vi "ForebrainMain.vi"() -> ()   [LabVIEW 2012]
uses:
  <vilib>/Utility/inputDevices.llb/closeKeyboard.vi
  <vilib>/Utility/inputDevices.llb/keyboardAcquire.vi
panel:
  out "IR Data":dbl
  in  "Send to XBEE":string
  out "bytes written":u32
  out "Sent from XBEE":string
  out "return count":u32
  out "XBEE Working":bool
  in  "FULL STOP":bool
  in  "PC Status":i32=1
  out "Port Rudder":i32
  out "Starboard Rudder":i32
  out "Port Motor":i32
  out "Starboard Motor":i32
  in  "VISA resource name":refnum<visa-resource-name>="COM6"
  in  "error in":errorcluster
  out "Base Station data rec'd":string
  out "Robot Stats":i32[](array[numeric])
  out "Buoy locations":cluster{"regular expression":string, i32, i32}[](array[cluster])
  in  "Tab Control":T1(tab)
  in  "End Rc Session":bool
  in  "Pan Camera":i32(slide)=1500 scale=500.0..2500.0
  in  "MANUAL \nOVERRIDE":bool
  out "Speed                    Balance":i32(knob) scale=-1000.0..1000.0
  in  "Step Size":i32=5
  in  "Rudders":i32(slide)=1500 scale=500.0..2500.0
  out "Port Speed":i32(knob) scale=1000.0..2000.0
  out "Starboard Speed":i32(knob) scale=1000.0..2000.0
  out "Obstacle Seen":bool
  in  "Launch":bool
  out "Forward":u8(slide) scale=0.0..100.0
  in  "Mission Selection":string(combo)
  out "Backward":u8(slide) scale=0.0..100.0
  # "This is the main VI.\n\nThis will allow you to debug the sensor system, remotely control the boat, and select a mission for the boat to run autonomously.  This code will connect to the base station, use the XBEE to connect to the boat, and use Labview as an interfacing platform with the boat.\n\nIf you have questions/comments/concerns, email Bill Warner or Victoria Preston (Olin)\n\nCreated:Feb 28, 2014\nRevised: Mar 9, 2014"
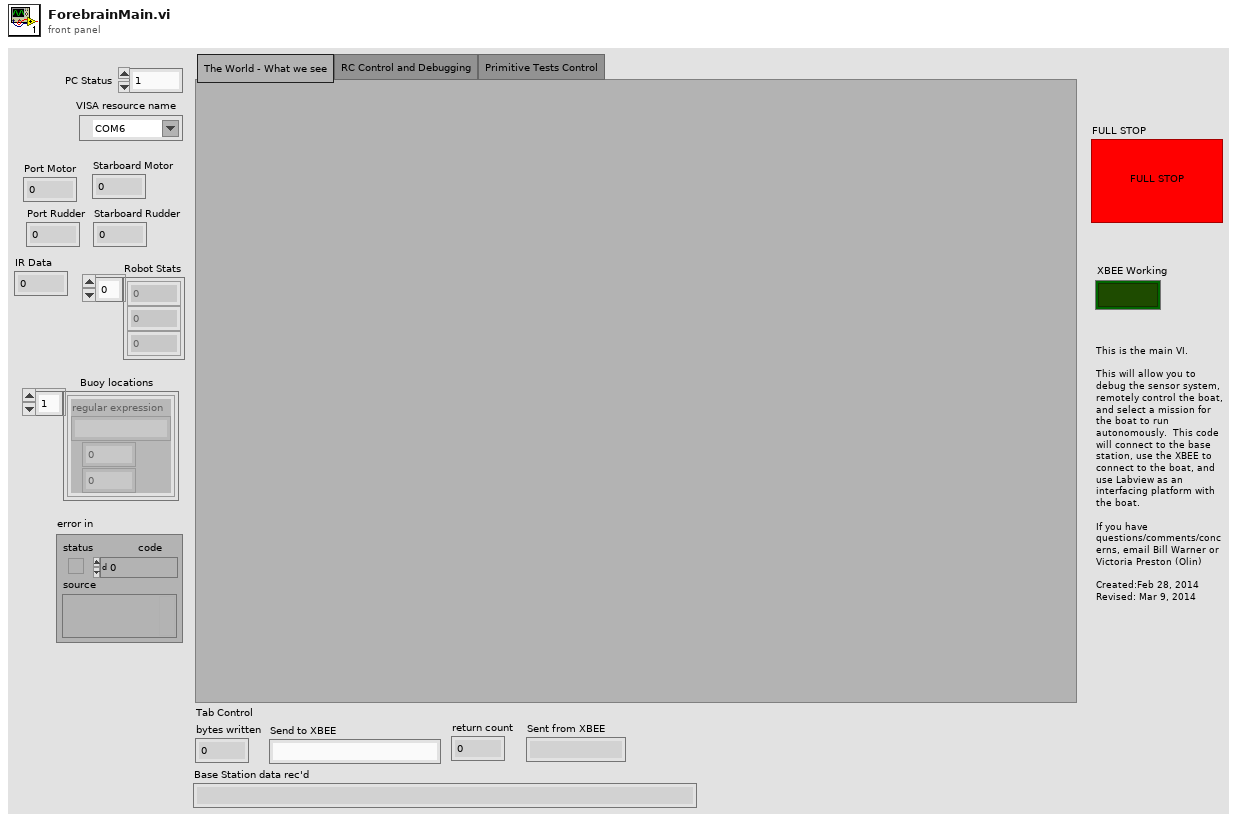
[diagram p1: front panel]
types:
  T1 = enum32{"The World - What we see", "RC Control and Debugging", "Primitive Tests Control"}
  T2 = enum16{"0", "1", "2", "3", "4", "5", "6", "7", "8", "9", "A", "B", "C", "D", "E", "F", "G", "H", "I", "J", "K", "L", "M", "N", "O", "P", "Q", "R", "S", "T", "U", "V", "W", "X", "Y", "Z", "F1", "F2", "F3", "F4", "F5", "F6", "F7", "F8", "F9", "F10", "F11", "F12", "F13", "F14", "F15", "ADD", "BACK", "BACKSLASH", "CAPITAL", "COMMA", "DECIMAL", "DELETE", "DIVIDE", "DOWN", "END", "EQUALS", "ESCAPE", "GRAVE (`)", "HOME", "INSERT", "LBRACKET", "LCONTROL", "LEFT", "L ALT", "LSHIFT", "LWIN", "MINUS", "MULTIPLY", "NEXT", "NUMLOCK", "NUMPAD_0", "NUMPAD_1", "NUMPAD_2", "NUMPAD_3", "NUMPAD_4", "NUMPAD_5", "NUMPAD_6", "NUMPAD_7", "NUMPAD_8", "NUMPAD_9", "PAUSE", "PERIOD", "PRIOR (PG UP)", "RBRACKET", "RCONTROL", "RETURN", "RIGHT", "R ALT", "RSHIFT", "RWIN", "SCROLL", "SEMICOLON", "SLASH", "SPACE", "SUBTRACT", "TAB", "UP", "ENTER (num pad)", "' (quote)"}[]
  T3 = enum16{"0", "1", "2", "3", "4", "5", "6", "7", "8", "9", "A", "B", "C", "D", "E", "F", "G", "H", "I", "J", "K", "L", "M", "N", "O", "P", "Q", "R", "S", "T", "U", "V", "W", "X", "Y", "Z", "F1", "F2", "F3", "F4", "F5", "F6", "F7", "F8", "F9", "F10", "F11", "F12", "F13", "F14", "F15", "ADD", "BACK", "BACKSLASH", "CAPITAL", "COMMA", "DECIMAL", "DELETE", "DIVIDE", "DOWN", "END", "EQUALS", "ESCAPE", "GRAVE (`)", "HOME", "INSERT", "LBRACKET", "LCONTROL", "LEFT", "L ALT", "LSHIFT", "LWIN", "MINUS", "MULTIPLY", "NEXT", "NUMLOCK", "NUMPAD_0", "NUMPAD_1", "NUMPAD_2", "NUMPAD_3", "NUMPAD_4", "NUMPAD_5", "NUMPAD_6", "NUMPAD_7", "NUMPAD_8", "NUMPAD_9", "PAUSE", "PERIOD", "PRIOR (PG UP)", "RBRACKET", "RCONTROL", "RETURN", "RIGHT", "R ALT", "RSHIFT", "RWIN", "SCROLL", "SEMICOLON", "SLASH", "SPACE", "SUBTRACT", "TAB", "UP", "ENTER (num pad)", "' (quote)"}
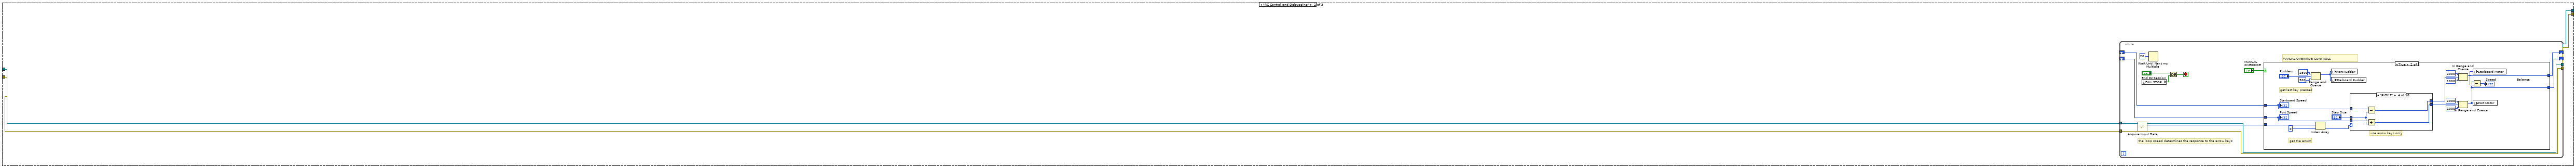
[diagram p3: hidden frame]
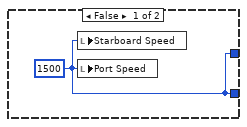
[diagram p4: hidden frame]
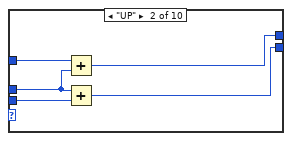
[diagram p6: hidden frame]
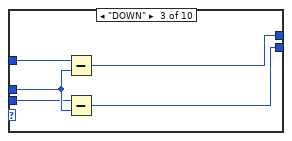
[diagram p7: hidden frame]
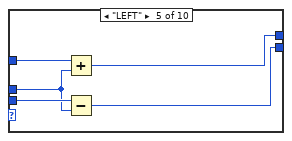
[diagram p8: hidden frame]
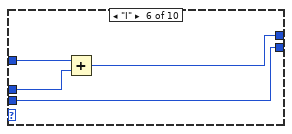
[diagram p9: hidden frame]
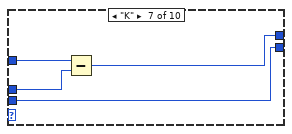
[diagram p10: hidden frame]
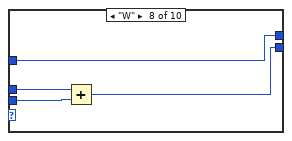
[diagram p11: hidden frame]
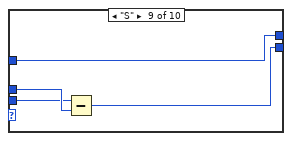
[diagram p12: hidden frame]
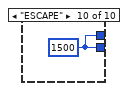
[diagram p13: hidden frame]
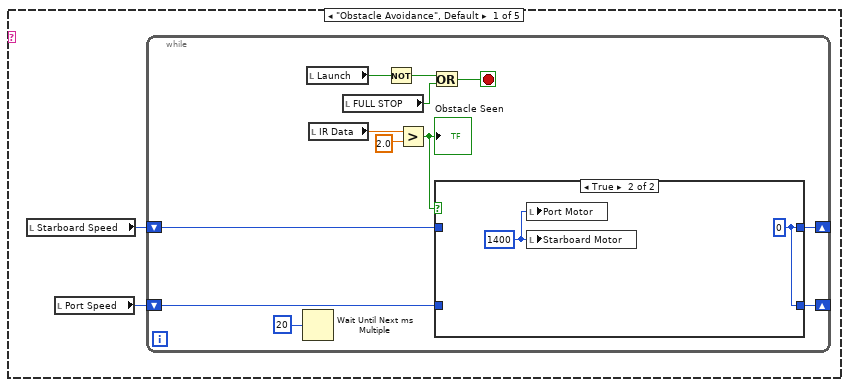
[diagram p15: hidden frame]
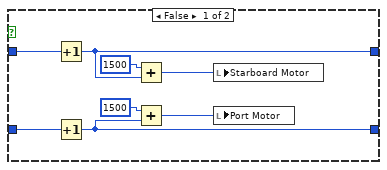
[diagram p16: hidden frame]
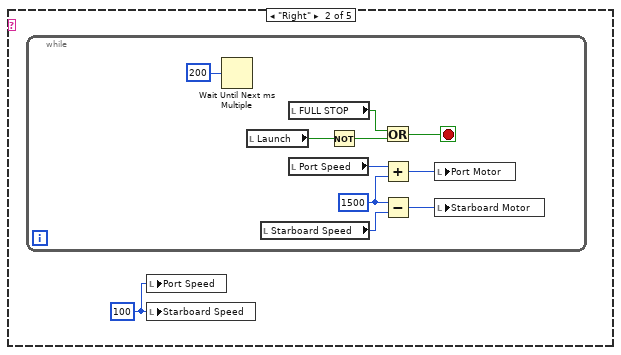
[diagram p17: hidden frame]
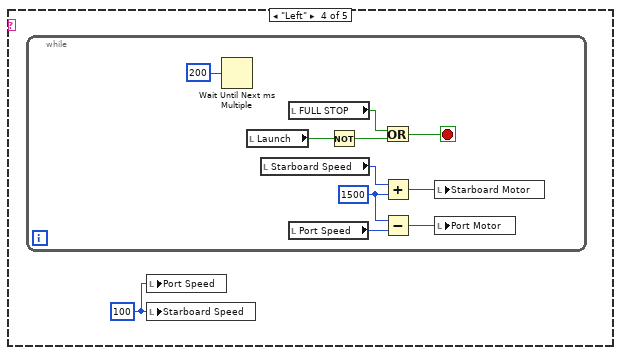
[diagram p18: hidden frame]
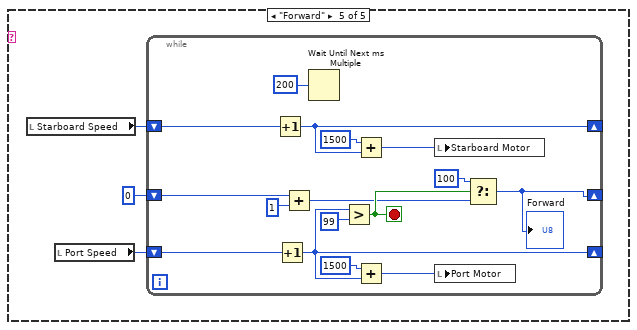
[diagram p19: hidden frame]
diagram:
  # "XBEE \nCOMMUNICATION\nBLOCK"
  n1 = flat-sequence {
    tunnel: [FALSE] -> _
    tunnel: [w12] -> w6
    tunnel: [w11] -> w5
    tunnel: [w10] -> w4
    tunnel: [w9] -> w3
    frame #0 {
      (unwired) 1500
      w19 = u16 61557  # Port
      # "Initializes Keyboard Override Controls"
      # "Initializes variables used in boat control"
      # "Initializes variables used in communication\nwith the on-board robot brain via XBEE."
      # "Initializes variables used in communication\nwith the pseudo-GPS computer and connects.\nThe GPS computer sends a string over UDP\nwhich is parsed into boat position and heading."
      # "Open UDP port to receive  boat location from Base staion"
      n2 = local write "Robot Stats"(i32[] [0, 0, 0, 0]) -> ()
      n3 = UDP Open(8:"error in", 9:25000 ("timeout ms (25000)"), 11:w19) -> ()  [unwired: 2 in, 3 out]
      n4 = call "XBEE Open.vi"("error in"=errorcluster {"status"=FALSE, "code"=0, "source"=""}, "VISA resource name"="VISA resource name") -> ("error out"=w11:errorcluster, "VISA resource name out"=w12:refnum<visa-resource-name>)
      n5 = call <vilib>:"Intialize Keyboard.vi"("error in (no error)"=errorcluster {"status"=FALSE, "code"=0, "source"=""}) -> ("error out"=w9:errorcluster, "device ID"=w10:refnum<k1>)  [unwired: 9 in]
    }
  }
  n6 = while {
    stop <- w31 stop-if-true
    # "Unpack XBEE broadcast"
    n7 = local read "Sent from XBEE"() -> (w27:string)
    n8 = String Subset(string=w27, offset (0)=3, length (rest)=5 ("length (rest)")) -> (substring=w28:string)
    n9 = Match Pattern(string=w27, regular expression="b", offset (0)=0) -> (after substring=w25:string)  [unwired: 3 out]
    n10 = Fract/Exp String To Number(string=w28) -> (number=w21:dbl)  [unwired: 3 in, 1 out]
    n11 = Fract/Exp String To Number(string=w25) -> (offset past number=w24:i32)  [unwired: 3 in, 1 out]
    n12 = local write "IR Data"(w21) -> ()
    n13 = Build Array(w24) -> (→"Robot Stats":i32[])
    n14 = local read "FULL STOP"() -> (w31:bool)
  }
  n15 = while {
    stop <- w61 stop-if-true
    # "Why this delay, Garland?"
    # "Prepare Command for XBEE transmission"
    # "Forms command string"
    n16 = Wait Until Next ms Multiple(millisecond multiple=u32 25) -> ()  [unwired: 1 out]
    n17 = local read "Starboard Rudder"() -> (w49:i32)
    n18 = local read "Starboard Motor"() -> (w58:i32)
    n19 = local read "Port Rudder"() -> (w46:i32)
    n20 = local read "Port Motor"() -> (w55:i32)
    n21 = local read "Pan Camera"() -> (w40:i32)
    n22 = local read "PC Status"() -> (w37:i32)
    n23 = Format Value(string ("")="S", format string="%4.0f", value (0)=w58) -> (output string=w53:string)
    n24 = Format Value(string ("")="P", format string="%4.0f", value (0)=w55) -> (output string=w52:string)
    n25 = Format Value(string ("")="R", format string="%4.0f", value (0)=w49) -> (output string=w45:string)
    n26 = Format Value(string ("")="L", format string="%4.0f", value (0)=w46) -> (output string=w44:string)
    n27 = Format Value(string ("")="P", format string="%4.0f", value (0)=w40) -> (output string=w35:string)
    n28 = Format Value(string ("")="H", format string="%4.0f", value (0)=w37) -> (output string=w34:string)
    n29 = Concatenate Strings("$C", w53, w52, w45, w44) -> (w36:string)
    n30 = Concatenate Strings(w36, w35, w34, "\n") -> (w41:string)
    n31 = local write "Send to XBEE"(w41) -> ()
    n32 = local read "FULL STOP"() -> (w61:bool)
  }
  n33 = while {
    tunnel: w6 -> [w75]
    tunnel: w5 -> [w74]
    tunnel: [w69] -> w8
    tunnel: [w68] -> w7
    shift-right: [w63] -> _
    shift-left: _ -> [w65]
    stop <- "FULL STOP" stop-if-true
    # "Why this delay, Garland?"
    # "XBEE Communication Loop"
    n34 = Not(x=w65) -> (.not. x?=w63:bool)
    "XBEE Working" <- w63
    n35 = Wait Until Next ms Multiple(millisecond multiple=200) -> ()  [unwired: 1 out]
    n36 = call "XBEE Send.vi"("error in (no error)"=w74, "String"="Send to XBEE", "VISA resource name"=w75) -> ("error out"=w71:errorcluster, "return count"=→"bytes written":u32, "VISA resource name out"=w72:refnum<visa-resource-name>)
    n37 = call "XBEE Hear.vi"("VISA resource name"=w72, "error in (no error)"=w71) -> ("VISA resource name out"=w69:refnum<visa-resource-name>, "String Received"=→"Sent from XBEE":string, "return count"=→"return count":u32, "error out"=w68:errorcluster)
  }
  n38 = while {
    tunnel: w4 -> [w81]
    tunnel: w3 -> [w80]
    tunnel: [w77] -> w2
    tunnel: [w76] -> w1
    stop <- w78 stop-if-true
    n39 = case shown="\"Primitive Tests Control\"" "Tab Control" {
      tunnel: w81 -> [_ w84 _]
      tunnel: w80 -> [_ w85 _]
      tunnel: [_ w83 _] -> w76
      tunnel: [_ w82 _] -> w77
      frame "The World - What we see", Default {
      }
      frame "RC Control and Debugging" {
        n40 = while {
          tunnel: [w99] -> w83
          tunnel: [w98] -> w82
          shift-right: [w93] -> _
          shift-left: _ -> [w95]
          shift-right: [w92] -> _
          shift-left: _ -> [w94]
          tunnel: w84 -> [w91]
          tunnel: w85 -> [w89]
          stop <- w88 stop-if-true
          # "MANUAL OVERRIDE CONTROLS"
          # "the loop speed determines the response to the arrow keys"
          n41 = call-poly <vilib>:"Acquire Input Data.vi"("device ID"=w91, "error in (no error)"=w89) -> ("device ID"=w98:refnum<k1>, "keys pressed"=w97:T2, "error out"=w99:errorcluster)  [unwired: 15 in]
          n42 = local read "FULL STOP"() -> (w86:bool)
          n43 = Wait Until Next ms Multiple(millisecond multiple=u32 20) -> ()  [unwired: 1 out]
          n44 = Or(x="End Rc Session", y=w86) -> (x .or. y?=w88:bool)
          n45 = case shown="True" "MANUAL \nOVERRIDE" {
            tunnel: w97 -> [_ w119]
            tunnel: w95 -> [_ w116]
            tunnel: w94 -> [_ w115]
            tunnel: [w100 w103] -> w93
            tunnel: [w100 w102] -> w92
            frame False {
              w100 = 1500
              n46 = local write "Starboard Speed"(w100) -> ()
              n47 = local write "Port Speed"(w100) -> ()
            }
            frame True {
              # "use arrow keys only"
              # "get the enum"
              # "get last key pressed"
              n48 = In Range and Coerce(upper limit=2500, x="Rudders", lower limit=500) -> (coerced(x)=w101:i32)  [unwired: 1 out]
              n49 = Index Array(array=w119, index=0) -> (element=w117:T3)
              n50 = local write "Port Rudder"(w101) -> ()
              n51 = local write "Starboard Rudder"(w101) -> ()
              n52 = case shown="\"RIGHT\"" w117 {
                tunnel: w116 -> [w121 w126 w131 w133 w138 w145 w147 w150 w154 _]
                tunnel: [w121 w125 w130 w134 w139 w144 w146 w150 w154 w158] -> w114
                tunnel: w115 -> [w120 w123 w128 w136 w140 w142 w149 w152 w156 _]
                tunnel: [w120 w122 w127 w135 w141 w142 w149 w151 w155 w158] -> w105
                tunnel: "Step Size" -> [_ w124 w129 w132 w137 w143 w148 w153 w157 _]
                frame "0", Default {
                }
                frame "UP" {
                  n53 = Add(x=w126, y=w124) -> (x+y=w125:i32)
                  n54 = Add(x=w124, y=w123) -> (x+y=w122:i32)
                }
                frame "DOWN" {
                  n55 = Subtract(x=w131, y=w129) -> (x-y=w130:i32)
                  n56 = Subtract(x=w128, y=w129) -> (x-y=w127:i32)
                }
                frame "RIGHT" {
                  n57 = Subtract(x=w133, y=w132) -> (x-y=w134:i32)
                  n58 = Add(x=w136, y=w132) -> (x+y=w135:i32)
                }
                frame "LEFT" {
                  n59 = Add(x=w138, y=w137) -> (x+y=w139:i32)
                  n60 = Subtract(x=w140, y=w137) -> (x-y=w141:i32)
                }
                frame "I" {
                  n61 = Add(x=w145, y=w143) -> (x+y=w144:i32)
                }
                frame "K" {
                  n62 = Subtract(x=w147, y=w148) -> (x-y=w146:i32)
                }
                frame "W" {
                  n63 = Add(x=w153, y=w152) -> (x+y=w151:i32)
                }
                frame "S" {
                  n64 = Subtract(x=w156, y=w157) -> (x-y=w155:i32)
                }
                frame "ESCAPE" {
                  w158 = 1500
                }
              }
              n65 = In Range and Coerce(upper limit=2000, x=w114, lower limit=1000) -> (coerced(x)=w103:i32)  [unwired: 1 out]
              n66 = In Range and Coerce(upper limit=2000, x=w105, lower limit=1000) -> (coerced(x)=w102:i32)  [unwired: 1 out]
              n67 = Subtract(x=w102, y=w103) -> (x-y=→"Speed                    Balance":i32)
              n68 = local write "Starboard Motor"(w103) -> ()
              n69 = local write "Port Motor"(w102) -> ()
              "Starboard Speed" <- w116
              "Port Speed" <- w115
            }
          }
        }
      }
      frame "Primitive Tests Control" {
        n70 = case shown="True" "Launch" {
          frame False {
          }
          frame True {
            n71 = flat-sequence {
              frame #0 {
                n72 = local write "Port Speed"(0) -> ()
                n73 = local write "Starboard Motor"(1500 ("Starboard Speed")) -> ()
                n74 = local write "Starboard Speed"(0 ("Starboard Speed")) -> ()
                n75 = local write "Port Motor"(1500 ("Port Motor")) -> ()
              }
              frame #1 {
                n76 = case shown="\"Backward\"" "Mission Selection" {
                  frame "Obstacle Avoidance", Default {
                    n77 = local read "Starboard Speed"() -> (w165:i32)
                    n78 = local read "Port Speed"() -> (w166:i32)
                    n79 = while {
                      shift-right: [w175] -> _
                      shift-left: w166 -> [w177]
                      shift-right: [w174] -> _
                      shift-left: w165 -> [w176]
                      stop <- w169 stop-if-true
                      n80 = Wait Until Next ms Multiple(millisecond multiple=u32 20) -> ()  [unwired: 1 out]
                      n81 = local read "Launch"() -> (w172:bool)
                      n82 = local read "IR Data"() -> (w167:dbl)
                      n83 = local read "FULL STOP"() -> (w170:bool)
                      n84 = Not(x=w172) -> (.not. x?=w171:bool)
                      n85 = Greater?(x=w167, y=2.0) -> (0:w168:bool)
                      "Obstacle Seen" <- w168
                      n86 = Or(x=w171, y=w170) -> (x .or. y?=w169:bool)
                      n87 = case shown="True" w168 {
                        tunnel: w177 -> [w182 _]
                        tunnel: w176 -> [w181 _]
                        tunnel: [w180 w187] -> w175
                        tunnel: [w179 w187] -> w174
                        frame False {
                          n88 = Increment(x=w181) -> (x+1=w179:i32)
                          n89 = Increment(x=w182) -> (x+1=w180:i32)
                          n90 = Add(x=1500, y=w179) -> (x+y=w183:i32)
                          n91 = Add(x=1500, y=w180) -> (x+y=w185:i32)
                          n92 = local write "Starboard Motor"(w183) -> ()
                          n93 = local write "Port Motor"(w185) -> ()
                        }
                        frame True {
                          w187 = 0
                          w188 = 1400
                          n94 = local write "Port Motor"(w188) -> ()
                          n95 = local write "Starboard Motor"(w188) -> ()
                        }
                      }
                    }
                  }
                  frame "Right" {
                    w189 = 100
                    n96 = while {
                      stop <- w195 stop-if-true
                      w192 = 1500
                      n97 = Wait Until Next ms Multiple(millisecond multiple=u32 200) -> ()  [unwired: 1 out]
                      n98 = local read "Launch"() -> (w198:bool)
                      n99 = local read "Starboard Speed"() -> (w191:i32)
                      n100 = local read "FULL STOP"() -> (w196:bool)
                      n101 = local read "Port Speed"() -> (w194:i32)
                      n102 = Not(x=w198) -> (.not. x?=w197:bool)
                      n103 = Or(x=w196, y=w197) -> (x .or. y?=w195:bool)
                      n104 = Add(x=w194, y=w192) -> (x+y=w193:i32)
                      n105 = Subtract(x=w192, y=w191) -> (x-y=w190:i32)
                      n106 = local write "Port Motor"(w193) -> ()
                      n107 = local write "Starboard Motor"(w190) -> ()
                    }
                    n108 = local write "Port Speed"(w189) -> ()
                    n109 = local write "Starboard Speed"(w189) -> ()
                  }
                  frame "Backward" {
                    n110 = local read "Starboard Speed"() -> (w201:i32)
                    n111 = local read "Port Speed"() -> (w202:i32)
                    n112 = while {
                      shift-right: [w208] -> _
                      shift-left: w202 -> [w218]
                      shift-right: [w204] -> _
                      shift-left: w201 -> [w217]
                      shift-right: [w203] -> _
                      shift-left: 0 -> [w213]
                      stop <- w215 stop-if-true
                      n113 = Increment(x=w217) -> (x+1=w204:i32)
                      n114 = Increment(x=w218) -> (x+1=w208:i32)
                      n115 = Add(x=w213, y=1) -> (x+y=w211:i32)
                      n116 = Wait Until Next ms Multiple(millisecond multiple=u32 200) -> ()  [unwired: 1 out]
                      n117 = Greater?(x=w208, y=99) -> (0:w215:bool)
                      n118 = Subtract(x=1500, y=w204) -> (x-y=w205:i32)
                      n119 = Subtract(x=1500, y=w208) -> (x-y=w207:i32)
                      n120 = local write "Starboard Motor"(w205) -> ()
                      n121 = local write "Port Motor"(w207) -> ()
                      n122 = Select(t=100, s=w215, f=w211) -> (s? t:f=w203:i32)
                      "Backward" <- w203
                    }
                  }
                  frame "Left" {
                    w219 = 100
                    n123 = while {
                      stop <- w225 stop-if-true
                      w222 = 1500
                      n124 = Wait Until Next ms Multiple(millisecond multiple=u32 200) -> ()  [unwired: 1 out]
                      n125 = local read "Launch"() -> (w228:bool)
                      n126 = local read "Starboard Speed"() -> (w224:i32)
                      n127 = local read "FULL STOP"() -> (w226:bool)
                      n128 = local read "Port Speed"() -> (w221:i32)
                      n129 = Not(x=w228) -> (.not. x?=w227:bool)
                      n130 = Or(x=w226, y=w227) -> (x .or. y?=w225:bool)
                      n131 = Add(x=w224, y=w222) -> (x+y=w223:i32)
                      n132 = Subtract(x=w222, y=w221) -> (x-y=w220:i32)
                      n133 = local write "Starboard Motor"(w223) -> ()
                      n134 = local write "Port Motor"(w220) -> ()
                    }
                    n135 = local write "Port Speed"(w219) -> ()
                    n136 = local write "Starboard Speed"(w219) -> ()
                  }
                  frame "Forward" {
                    n137 = local read "Starboard Speed"() -> (w231:i32)
                    n138 = local read "Port Speed"() -> (w232:i32)
                    n139 = while {
                      shift-right: [w238] -> _
                      shift-left: w232 -> [w248]
                      shift-right: [w234] -> _
                      shift-left: w231 -> [w247]
                      shift-right: [w233] -> _
                      shift-left: 0 -> [w243]
                      stop <- w245 stop-if-true
                      n140 = Increment(x=w247) -> (x+1=w234:i32)
                      n141 = Increment(x=w248) -> (x+1=w238:i32)
                      n142 = Add(x=w243, y=1) -> (x+y=w241:i32)
                      n143 = Wait Until Next ms Multiple(millisecond multiple=u32 200) -> ()  [unwired: 1 out]
                      n144 = Greater?(x=w238, y=99) -> (0:w245:bool)
                      n145 = Add(x=1500, y=w234) -> (x+y=w235:i32)
                      n146 = Add(x=1500, y=w238) -> (x+y=w237:i32)
                      n147 = local write "Starboard Motor"(w235) -> ()
                      n148 = local write "Port Motor"(w237) -> ()
                      n149 = Select(t=100, s=w245, f=w241) -> (s? t:f=w233:i32)
                      "Forward" <- w233
                    }
                  }
                }
              }
              frame #2 {
                w249 = 0
                w250 = 1500 ("Starboard Motor")
                n150 = local write "Launch"(FALSE) -> ()
                n151 = local write "Port Motor"(w250) -> ()
                n152 = local write "Starboard Motor"(w250) -> ()
                n153 = local write "Port Speed"(w249) -> ()
                n154 = local write "Starboard Speed"(w249) -> ()
              }
            }
          }
        }
      }
    }
    n155 = local read "FULL STOP"() -> (w78:bool)
  }
  n156 = call "XBEE Close.vi"("error in (no error)"=w7, "VISA resource name"=w8) -> ()
  n157 = call-poly <vilib>:"Close Input Device.vi"("error in (no error)"=w1, "device ID"=w2) -> ()  [unwired: 8 in, 1 out]
